vi "Radio Get Energy Per CM2.vi"(7 "a_inttime":dbl, 8 "error in (no error)":errorcluster, 9 "a_endwav":dbl, 10 "a_startwav":dbl, 11 "a_data":dbl[](array[numeric])) -> (0 "error out":errorcluster, 2 "function return":i16, 3 "a_data out":dbl[](array[numeric]), 4 "a_integral out":dbl)   [LabVIEW 2013, in "AvaSpec.lvlib" / "AVSirrad.lvlib"]
doc: "DLL_API short int __stdcall Radio_GetEnergyPerCM2\n(\n DataType *a_data,\n double a_startwav,\n double a_endwav,\n double a_inttime,\n double *a_integral\n);"
uses:
  AVSirrad.lvlib
  AVSirrad.dll
panel:
  in  "a_integral":dbl
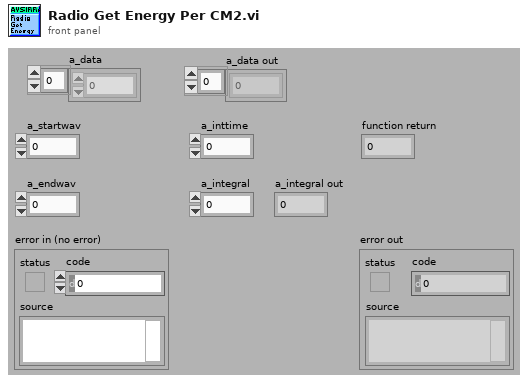
[diagram p1: front panel]
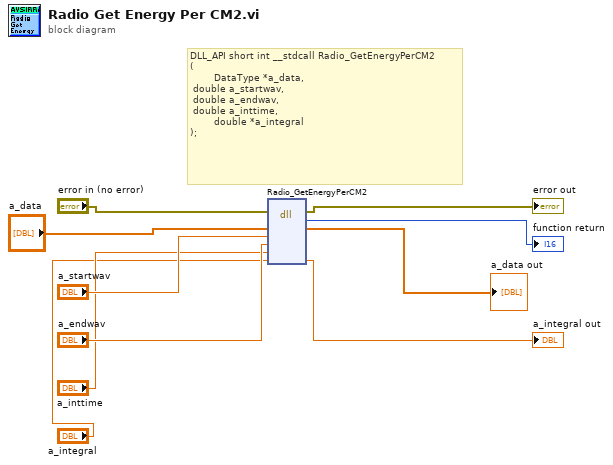
[diagram p0: block diagram]
diagram:
  # "DLL_API short int __stdcall Radio_GetEnergyPerCM2\n(\n        DataType *a_data,\n\tdouble a_startwav,\n\tdouble a_endwav,\n\tdouble a_inttime,\n        double *a_integral\n);"
  n1 = dll-call lib="C:/Users/dhstuart/Dropbox/CLTC/avantesSpectrometer/Libraries/IRRAD-DLL/AVSirrad.*" fn="Radio_GetEnergyPerCM2"(error in="error in (no error)", "a_data"="a_data", "a_startwav"="a_startwav", "a_endwav"="a_endwav", "a_inttime"="a_inttime", "a_integral"="a_integral") -> (error out=→"error out":errorcluster, "return type"=→"function return":i16, "a_data"=→"a_data out":dbl[], "a_integral"=→"a_integral out":dbl)  [unwired: 5 in, 1 out]
